vi "WriteParameters.vi"(0 "Data Save Directory:":path=path "C:/Data/test", 1 "Detectors Select":enum32{"4 Detectors", "8 Detectors"}(ring), 2 "Raster":bool, 6 "File Name:":string="tst8", 8 "X steps":u32, 10 "Y steps":u32, 12 "X increment (dx)":dbl, 14 "Y increment (dy)":dbl) -> (19 "error out":errorcluster)   [LabVIEW 2011]
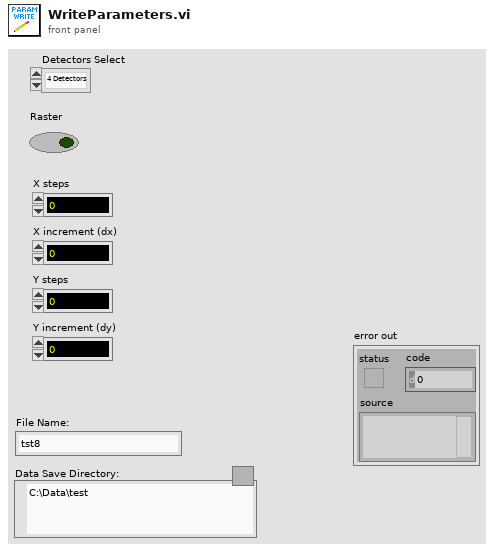
[diagram p1: front panel]
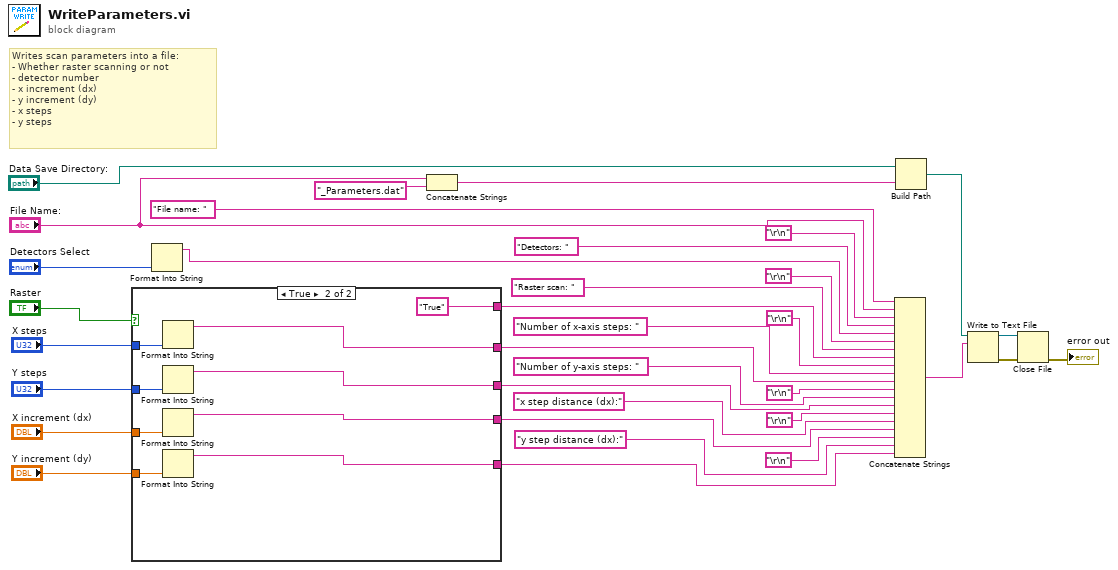
[diagram p0: block diagram]
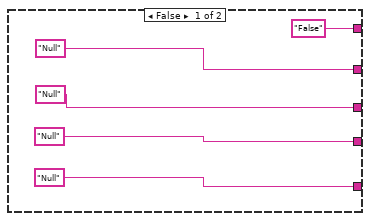
[diagram p2: hidden frame]
diagram:
  # "Writes scan parameters into a file:\n- Whether raster scanning or not \n- detector number\n- x increment (dx)\n- y increment (dy)\n- x steps\n- y steps"
  n1 = case shown="True" "Raster" {
    tunnel: "X steps" -> [_ w48]
    tunnel: "Y steps" -> [_ w47]
    tunnel: "X increment (dx)" -> [_ w46]
    tunnel: "Y increment (dy)" -> [_ w45]
    tunnel: ["Null" w44] -> w25
    tunnel: ["Null" w43] -> w22
    tunnel: ["Null" w42] -> w19
    tunnel: ["Null" w41] -> w1
    tunnel: ["False" "True"] -> w28
    frame False {
    }
    frame True {
      n2 = Format Into String(w48) -> (resulting string=w44:string)  [unwired: 3 in, 1 out]
      n3 = Format Into String(w47) -> (resulting string=w43:string)  [unwired: 3 in, 1 out]
      n4 = Format Into String(w46) -> (resulting string=w42:string)  [unwired: 3 in, 1 out]
      n5 = Format Into String(w45) -> (resulting string=w41:string)  [unwired: 3 in, 1 out]
    }
  }
  n6 = Format Into String("Detectors Select") -> (resulting string=w16:string)  [unwired: 3 in, 1 out]
  n7 = Concatenate Strings("File Name:", "_Parameters.dat") -> (w9:string)
  n8 = Concatenate Strings("File name: ", "File Name:", "\r\n", "Detectors: ", w16, "\r\n", "Raster scan: ", w28, "\r\n", "Number of x-axis steps: ", w25, "\r\n", "Number of y-axis steps: ", w22, "\r\n", "x step distance (dx):", w19, "\r\n", "y step distance (dx):", w1) -> (w7:string)
  n9 = Build Path(base path="Data Save Directory:", name or relative path=w9) -> (appended path=w8:path)
  n10 = Write to Text File(file (use dialog)=w8, text=w7) -> (refnum out=w6:refnum<file>, error out=w5:errorcluster)  [unwired: 2 in, 1 out]
  n11 = Close File(refnum=w6, error in=w5) -> (error out=→"error out":errorcluster)  [unwired: 1 out]
